vi "XY Graph Plot ASCII File Format Dialog.vi"(8 "error in (no error)":errorcluster) -> (0 "error out":errorcluster, 3 "Plot Format Information":T1, 4 "OK":bool)   [LabVIEW 2021, in "XY Graph Add-Ons.lvlib"]
doc: "Displays a standard dialog box that prompts users to enter information, such as a user name and password.\n--------------------\n\nThis Express VI is configured as follows:\n\nMessage to Display to the User:Define File Format\nThe inputs are: \nNumber: Number of Lines to Skip:\nCheckbox: Header Line?\nText Entry Box: Separator:"
uses:
  XY Graph Add-Ons.lvlib
  XY Graph Plot Format Information.ctl
panel:
  in  "User-Defined Separator":string
  in  "Abscissa Start":dbl
  in  "Abscissa Step":dbl
  in  "Abscissa Column?":bool
  in  "Separator":string(combo)="Tab" caption="Separator:"
  in  "Column Header Line?":bool caption="Header Line?"
  in  "Number of Lines to Skip":i32 caption="Number of Lines to Skip:"
  out "String":string="Define Data Format:"
  in  "Cancel":bool
  in  "OK2":bool
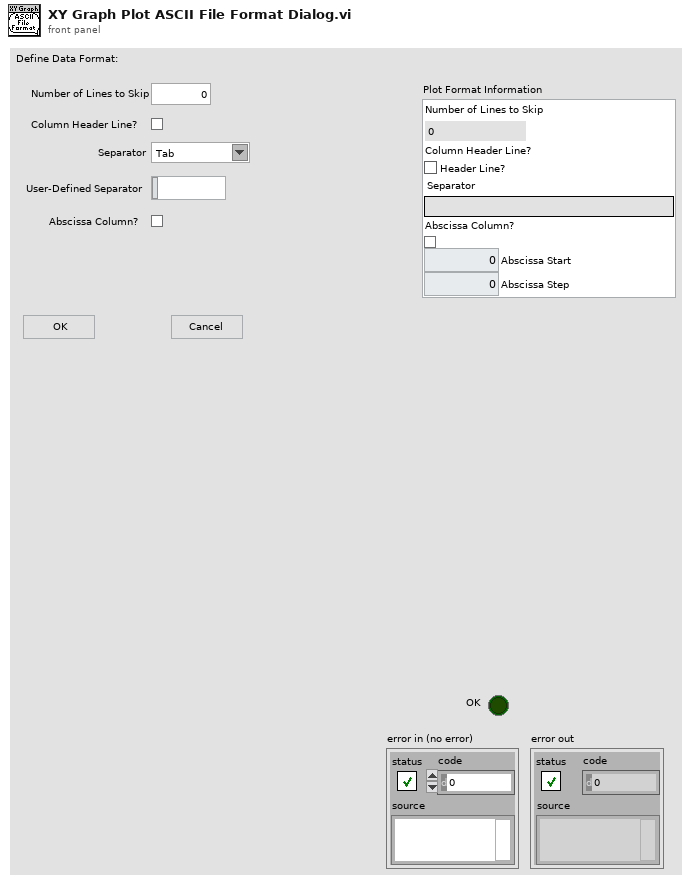
[diagram p1: front panel]
types:
  T1 = typedef "XY Graph Add-Ons.lvlib/XY Graph Plot Format Information.ctl" = cluster{"Number of Lines to Skip":i32, "Column Header Line?":bool, "Separator":string, "Abscissa Column?":bool, "Abscissa Start":dbl, "Abscissa Step":dbl}
  T2 = cluster{"Input Name":string, "Input Data Type":i32}[]
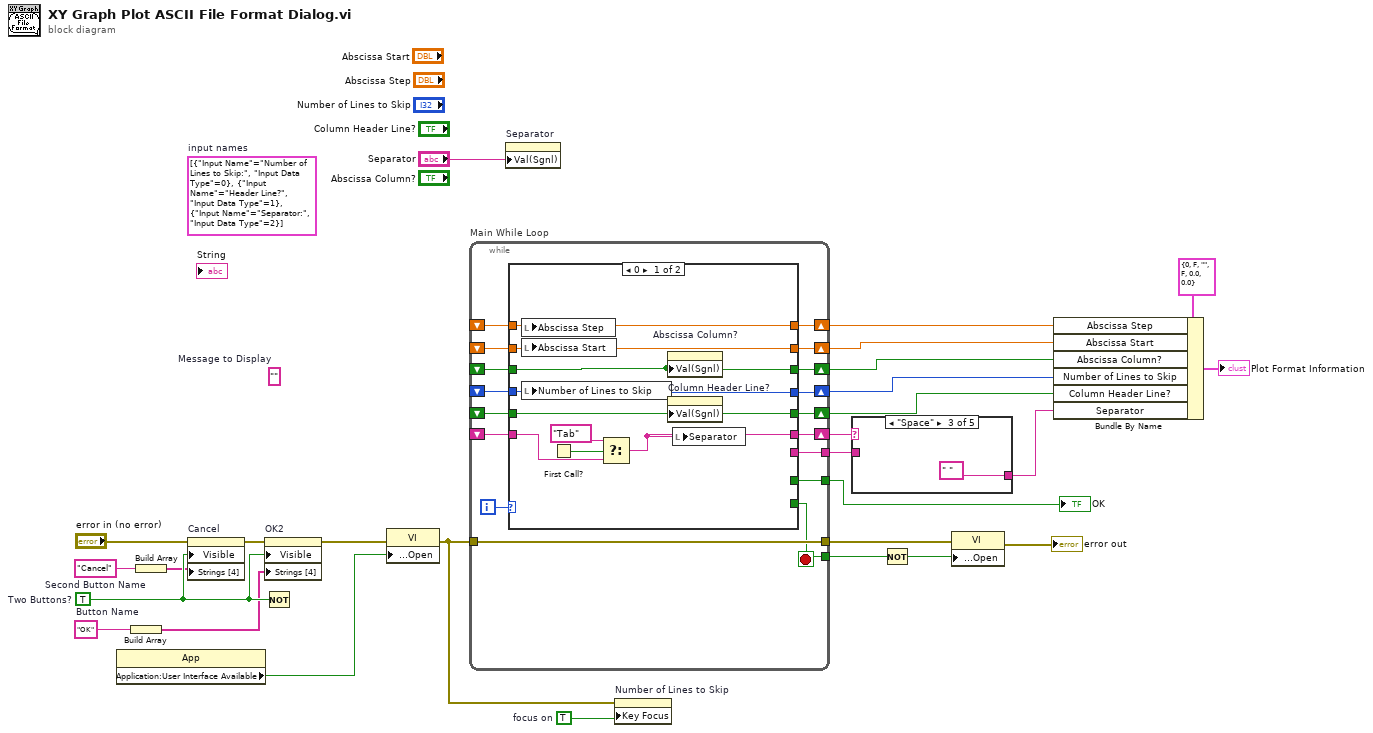
[diagram p0: block diagram]
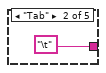
[diagram p3: hidden frame]
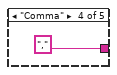
[diagram p4: hidden frame]
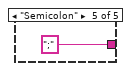
[diagram p5: hidden frame]
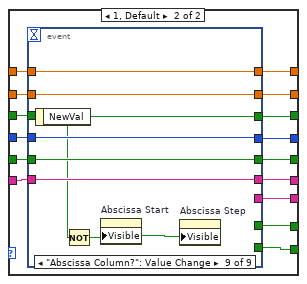
[diagram p6: hidden frame]
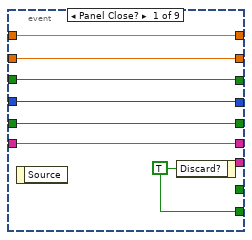
[diagram p7: hidden frame]
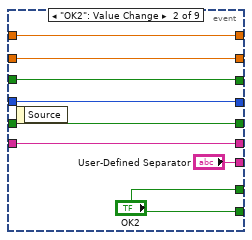
[diagram p8: hidden frame]
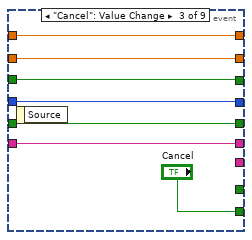
[diagram p9: hidden frame]
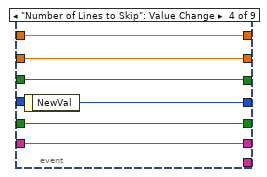
[diagram p10: hidden frame]
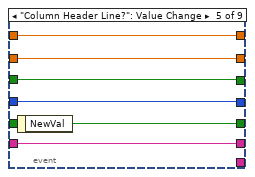
[diagram p11: hidden frame]
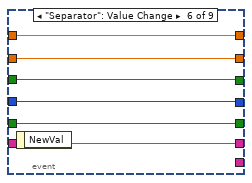
[diagram p12: hidden frame]
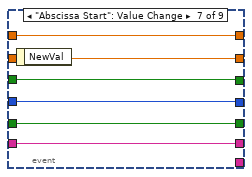
[diagram p13: hidden frame]
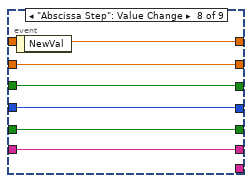
[diagram p14: hidden frame]
diagram:
  w15 = TRUE  # focus on
  (unwired) T2 [{"Input Name"="Number of Lines to Skip:", "Input Data Type"=0}, {"Input Name"="Header Line?", "Input Data Type"=1}, {"Input Name"="Separator:", "Input Data Type"=2}]  # input names
  w22 = "Cancel"  # Second Button Name
  w20 = "OK"  # Button Name
  (unwired) ""  # Message to Display
  w27 = TRUE  # Two Buttons?
  n1 = property class="App"() -> ("Application:User Interface Available"=w13:bool)  [unwired: 2 in, 2 out]
  n2 = Build Array(w20) -> (w21:string[])
  n3 = Build Array(w22) -> (w23:string[])
  n4 = property on="Cancel" class="Bool"(error in="error in (no error)", "Visible"=w27, "Strings [4]"=w23) -> (error out=w26:errorcluster)  [unwired: 1 in, 1 out]
  n5 = Not(x=w27) -> ()  [unwired: 1 out]
  n6 = property on="OK2" class="Bool"(error in=w26, "Visible"=w27, "Strings [4]"=w21) -> (error out=w14:errorcluster)  [unwired: 1 in, 1 out]
  n7 = property class="VI"(error in=w14, "Front Panel Window:Open"=w13) -> (error out=w19:errorcluster)  [unwired: 1 in, 1 out]
  n8 = while "Main While Loop" {
    tunnel: [w43] -> w24
    tunnel: w19 -> [w44]
    tunnel: [w44] -> w17
    tunnel: [w42] -> w12
    shift-right: [w40] -> w3
    shift-left: _ -> [w39]
    shift-right: [w38] -> w2
    shift-left: _ -> [w37]
    shift-right: [w36] -> w11
    shift-left: _ -> [w35]
    shift-right: [w33] -> w4
    shift-left: _ -> [w34]
    shift-right: [w32] -> w5
    shift-left: _ -> [w31]
    shift-right: [w30] -> w6
    shift-left: _ -> [w29]
    tunnel: [w28] -> w9
    i -> [w41]
    stop <- w43 stop-if-true
    n9 = case shown="0" w41 {
      tunnel: [_ w68] -> w43
      tunnel: [_ w67] -> w42
      tunnel: [w53 w66] -> w40
      tunnel: w39 -> [w53 w60]
      tunnel: [w50 w65] -> w38
      tunnel: w37 -> [w50 w61]
      tunnel: [w46 w64] -> w36
      tunnel: w35 -> [w48 w62]
      tunnel: w34 -> [w45 w59]
      tunnel: [w45 w63] -> w33
      tunnel: [w52 w58] -> w32
      tunnel: w31 -> [w52 w57]
      tunnel: [w51 w56] -> w30
      tunnel: w29 -> [w51 w55]
      tunnel: [_ w54] -> w28
      frame 0 {
        n10 = local write "Abscissa Step"(w51) -> ()
        n11 = local write "Abscissa Start"(w52) -> ()
        n12 = local write "Number of Lines to Skip"(w53) -> ()
        n13 = First Call?() -> (First Call?: T/F=w49:bool)
        n14 = Select(t="Tab" ("Separator"), s=w49, f=w48) -> (s? t:f=w46:string)
        n15 = property on="Abscissa Column?" class="Bool (strict)"("Val(Sgnl)"=w45) -> ()  [unwired: 2 in, 2 out]
        n16 = property on="Column Header Line?" class="Bool (strict)"("Val(Sgnl)"=w50) -> ()  [unwired: 2 in, 2 out]
        n17 = local write "Separator"(w46) -> ()
      }
      frame 1, Default {
        n18 = event shown="[8] \"Abscissa Column?\": Value Change" {
          selector: _ -> [_ _ _ _ _ _ _ _ _]
          dyn-events: _ -> [_ _ _ _ _ _ _ _ _]
          timeout: _ -> [_ _ _ _ _ _ _ _ _]
          tunnel: [w75 "OK2" "Cancel" _ _ _ _ _ _] -> w68
          tunnel: [_ "OK2" _ _ _ _ _ _ _] -> w67
          tunnel: [w72 w80 w87 w96 w100 w106 w113 w119 w125] -> w66
          tunnel: [w73 w81 w88 w94 w102 w107 w114 w120 w126] -> w65
          tunnel: [w74 w82 w89 w95 w101 w108 w109 w115 w127] -> w64
          tunnel: [w71 w79 w86 w93 w99 w105 w112 w118 w124] -> w63
          tunnel: w62 -> [w74 w82 w89 w95 w101 _ w109 w115 w127]
          tunnel: w61 -> [w73 w81 w88 w94 _ w107 w114 w120 w126]
          tunnel: w60 -> [w72 w80 w87 _ w100 w106 w113 w119 w125]
          tunnel: w59 -> [w71 w79 w86 w93 w99 w105 w112 w118 _]
          tunnel: [w70 w78 w85 w92 w98 w104 w111 w116 w122] -> w58
          tunnel: w57 -> [w70 w78 w85 w92 w98 w104 _ w116 w122]
          tunnel: [w69 w77 w84 w91 w97 w103 w110 w117 w121] -> w56
          tunnel: w55 -> [w69 w77 w84 w91 w97 w103 w110 _ w121]
          tunnel: [_ "User-Defined Separator" _ _ _ _ _ _ _] -> w54
          event Panel Close? {
            w75 = TRUE ("Discard?")
            n19 = event-data() -> ()  [unwired: 1 in, 1 out]
            n20 = event-data("Discard?"=w75) -> ()  [unwired: 1 in, 1 out]
          }
          event "OK2": Value Change {
            n21 = event-data() -> ()  [unwired: 1 in, 1 out]
          }
          event "Cancel": Value Change {
            n22 = event-data() -> ()  [unwired: 1 in, 1 out]
          }
          event "Number of Lines to Skip": Value Change {
            n23 = event-data() -> ("NewVal"=w96:i32)  [unwired: 1 in]
          }
          event "Column Header Line?": Value Change {
            n24 = event-data() -> ("NewVal"=w102:bool)  [unwired: 1 in]
          }
          event "Separator": Value Change {
            n25 = event-data() -> ("NewVal"=w108:string)  [unwired: 1 in]
          }
          event "Abscissa Start": Value Change {
            n26 = event-data() -> ("NewVal"=w111:dbl)  [unwired: 1 in]
          }
          event "Abscissa Step": Value Change {
            n27 = event-data() -> ("NewVal"=w117:dbl)  [unwired: 1 in]
          }
          event "Abscissa Column?": Value Change {
            n28 = event-data() -> ("NewVal"=w124:bool)  [unwired: 1 in]
            n29 = Not(x=w124) -> (.not. x?=w123:bool)
            n30 = property on="Abscissa Start" class="DigNum (strict)"("Visible"=w123) -> ()  [unwired: 2 in, 2 out]
            n31 = property on="Abscissa Step" class="DigNum (strict)"("Visible"=w123) -> ()  [unwired: 2 in, 2 out]
          }
        }
      }
    }
  }
  "OK" <- w12
  n32 = property on="Separator" class="CmbBox"("Val(Sgnl)"="Separator") -> ()  [unwired: 2 in, 2 out]
  n33 = property on="Number of Lines to Skip" class="DigNum (strict)"(error in=w19, "Key Focus"=w15) -> ()  [unwired: 1 in, 2 out]
  n34 = case shown="\"Space\"" w11 {
    tunnel: [w128 "\t" " " "," ";"] -> w1
    tunnel: w9 -> [w128 _ _ _ _]
    frame "User-Defined", Default {
    }
    frame "Tab" {
    }
    frame "Space" {
    }
    frame "Comma" {
    }
    frame "Semicolon" {
    }
  }
  n35 = Not(x=w24) -> (.not. x?=w25:bool)
  n36 = property class="VI"(error in=w17, "Front Panel Window:Open"=w25) -> (error out=→"error out":errorcluster)  [unwired: 1 in, 1 out]
  n37 = Bundle By Name(cluster=T1 {"Number of Lines to Skip"=0, "Column Header Line?"=FALSE, "Separator"="", "Abscissa Column?"=FALSE, "Abscissa Start"=0.0, "Abscissa Step"=0.0} ("Plot Format Information"), "Abscissa Step"=w6, "Abscissa Start"=w5, "Abscissa Column?"=w4, "Number of Lines to Skip"=w3, "Column Header Line?"=w2, "Separator"=w1) -> (→"Plot Format Information":T1)
